vi "Query Alarm Status.vi"(8 "error in":errorcluster, 11 "6700 in":refnum<class "6700.lvclass">) -> (0 "error out":errorcluster, 2 "Alarm":bool, 3 "6700 out":refnum<class "6700.lvclass">)   [LabVIEW 2018, in "6700.lvlib" / "6700.lvclass"]
uses:
  6700.lvclass
  6700.lvclass/6700.ctl
  builds/Power_Supply.lvlibp/Power Supply.lvclass
  <instrlib>/Agilent N6700 Series/Agilent N6700 Series.lvlib
  C:/Users/Ron.Dexter.LUMINARTECH/Desktop/builds/Power_Supply.lvlibp/Power Supply.lvclass
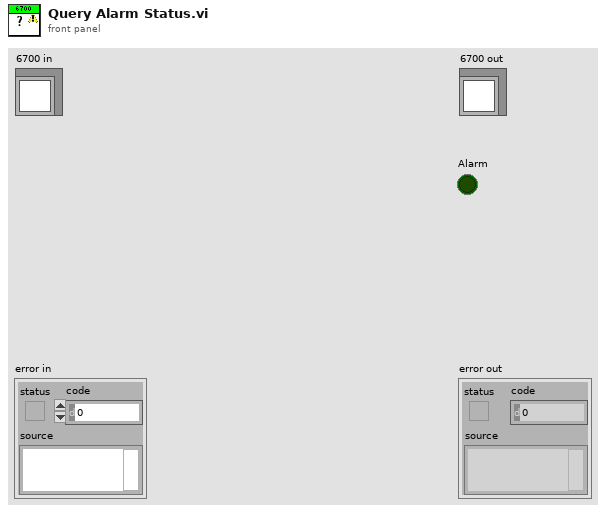
[diagram p1: front panel]
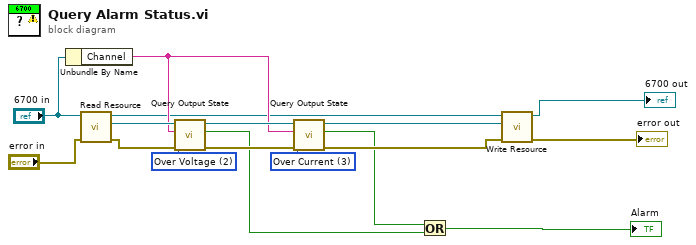
[diagram p0: block diagram]
diagram:
  w13 = 3 items=["Constant Voltage"=0, "Constant Current"=1, "Unregulated"=4, "Over Voltage"=2, "Over Current"=3] ("Output State (0: Constant Voltage)")
  w14 = 2 items=["Constant Voltage"=0, "Constant Current"=1, "Unregulated"=4, "Over Voltage"=2, "Over Current"=3] ("Output State (0: Constant Voltage)")
  n1 = Unbundle By Name("6700 in") -> ("Channel"=w9:string)
  n2 = call "Read Resource.vi"("error in"="error in", "Power Supply in"="6700 in") -> ("error out"=w10:errorcluster, "Resource"=w15:refnum<visa-resource-name>, "Power Supply out"=w8:refnum<class "6700.lvclass">)  [unwired: 7 in]
  n3 = call <instrlib>:"Query Output State.vi"("error in (no error)"=w10, "Output State (0: Constant Voltage)"=w14, "Channel Name (1)"=w9, "VISA resource name"=w15) -> ("error out"=w11:errorcluster, "In State"=w2:bool, "VISA resource name out"=w12:refnum<visa-resource-name>)  [unwired: 5 in]
  n4 = call <instrlib>:"Query Output State.vi"("error in (no error)"=w11, "Output State (0: Constant Voltage)"=w13, "Channel Name (1)"=w9, "VISA resource name"=w12) -> ("error out"=w6:errorcluster, "In State"=w3:bool, "VISA resource name out"=w7:refnum<visa-resource-name>)  [unwired: 5 in]
  n5 = Or(x=w3, y=w2) -> (x .or. y?=→"Alarm":bool)
  n6 = call "Write Resource.vi"("error in"=w6, "Resource"=w7, "Power Supply in"=w8) -> ("error out"=→"error out":errorcluster, "Power Supply out"=→"6700 out":refnum<class "6700.lvclass">)  [unwired: 7 in]
